vi "Epoxy_Save.vi"(6 "Valve A, B":dbl[](array[numeric]), 7 "Labels":string[](array[string])=["Time", "Box 1 [amps]", "Box 2 [amps]", "Flk 3 [amps]", "Flk 4 [amps]", "Flk 5 [amps]", "VAC"], 8 "error in (no error)":errorcluster, 9 "Int Done?":bool, 10 "Data Cluster":T2, 11 "Cluster":T1) -> (0 "error out":errorcluster)   [LabVIEW 2020]
uses:
  controls/UI Data.ctl
  DAQLoop_Typedef.ctl
  controls/SaveTimer.ctl
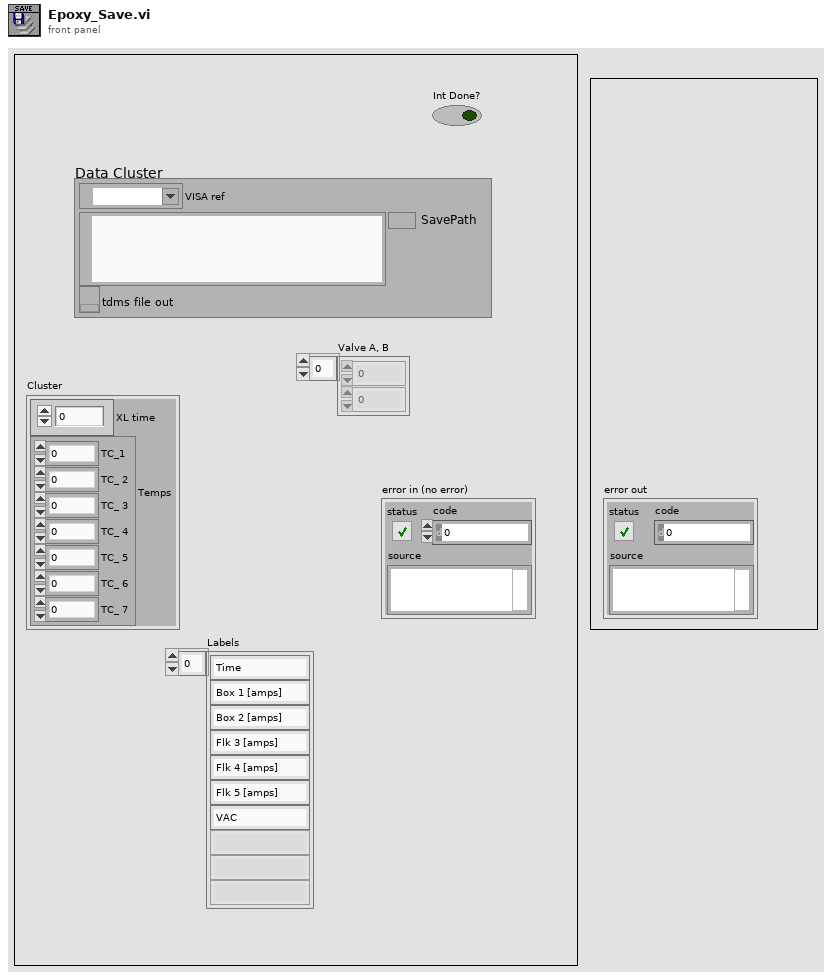
[diagram p1: front panel]
types:
  T1 = typedef "DAQLoop_Typedef.ctl" = cluster{"XL time":dbl, "Temps":cluster{"TC_1":dbl, "TC_ 2":dbl, "TC_ 3":dbl, "TC_ 4":dbl, "TC_ 5":dbl, "TC_ 6":dbl, "TC_ 7":dbl}}
  T2 = typedef "UI Data.ctl" = cluster{"VISA ref":refnum<visa-resource-name>, "SavePath":path, "tdms file out":refnum<k34>}
  T3 = typedef "SaveTimer.ctl" = enum16{"Start Save", "StartInterval", "UpdateInterval", "Check"}
  T4 = cluster{"TC_1":dbl, "TC_ 2":dbl, "TC_ 3":dbl, "TC_ 4":dbl, "TC_ 5":dbl, "TC_ 6":dbl, "TC_ 7":dbl}
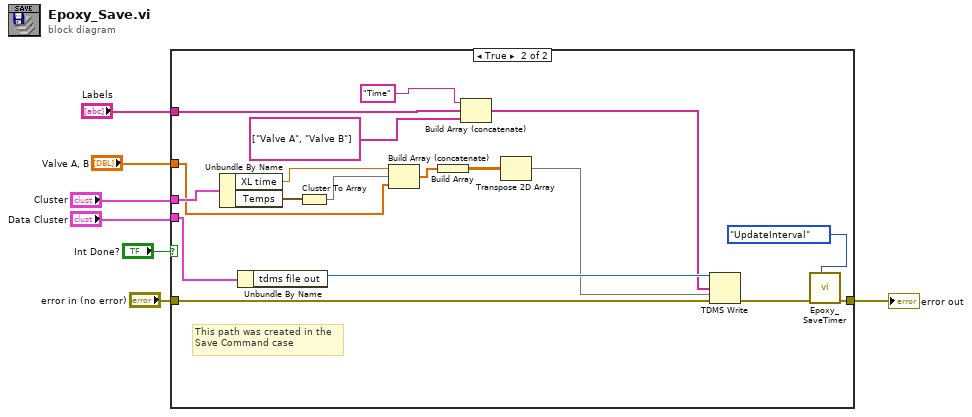
[diagram p0: block diagram]
diagram:
  n1 = case shown="True" "Int Done?" {
    tunnel: "Cluster" -> [_ w22]
    tunnel: "error in (no error)" -> [w8 w21]
    tunnel: "Data Cluster" -> [_ w26]
    tunnel: [w8 w25] -> w7
    tunnel: "Labels" -> [_ w15]
    tunnel: "Valve A, B" -> [_ w9]
    frame False {
    }
    frame True {
      # "This path was created in the\nSave Command case"
      n2 = Unbundle By Name(w22) -> ("XL time"=w19:dbl, "Temps"=w12:T4)
      n3 = Unbundle By Name(w26) -> ("tdms file out"=w20:refnum<k34>)
      n4 = Cluster To Array(cluster=w12) -> (array=w11:dbl[])
      n5 = Build Array (concatenate)(w19, w11, w9) -> (w18:dbl[])
      n6 = Build Array(w18) -> (w17:dbl[][])
      n7 = Build Array (concatenate)("Time", w15, string[] ["Valve A", "Valve B"] ("array")) -> (w13:string[])
      n8 = Transpose 2D Array(2D array=w17) -> (transposed array=w16:dbl[][])
      n9 = TDMS Write(0:w20, 7:w13, 9:w16, 11:w21) -> (15:w23:errorcluster)  [unwired: 2 in, 3 out]
      n10 = call "Epoxy_SaveTimer.vi"("Enum"=SaveTimer."UpdateInterval", "error in (no error)"=w23) -> ("error out"=w25:errorcluster)  [unwired: 6 in, 3 out]
    }
  }
  "error out" <- w7
